vi "Smooth All Planes.vi"(8 "error in (no error)":errorcluster, 11 "Images":T1) -> (0 "error out":errorcluster, 3 "Images":T1)   [LabVIEW 2015]
uses:
  controls/Images.ctl
  <vilib>/vision/Image Controls.llb/IMAQ Image.ctl
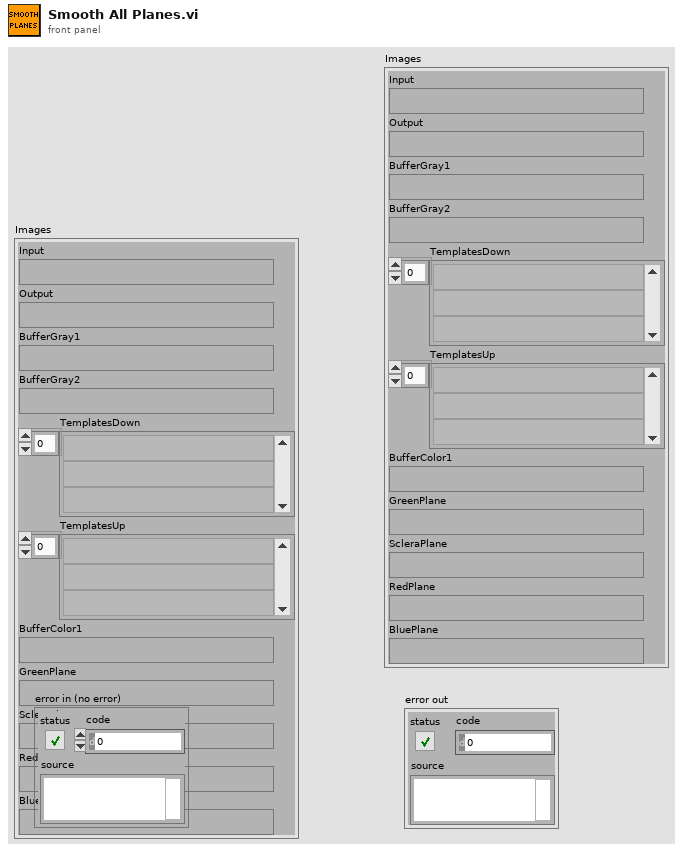
[diagram p1: front panel]
types:
  T1 = typedef "Images.ctl" = cluster{"Input":T2, "Output":T2, "BufferGray1":T2, "BufferGray2":T2, "TemplatesDown":T2[], "TemplatesUp":T2[], "BufferColor1":T2, "GreenPlane":T2, "ScleraPlane":T2, "RedPlane":T2, "BluePlane":T2}
  T2 = typedef "IMAQ Image.ctl" = refnum<image>
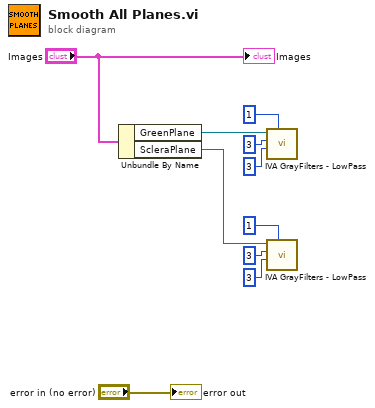
[diagram p0: block diagram]
diagram:
  n1 = Unbundle By Name("Images") -> ("GreenPlane"=w3:T2, "ScleraPlane"=w2:T2)
  n2 = call <vilib>:"IVA GrayFilters - LowPass.vi"("Tolerance"=1, "Filter size Y"=3, "Filter size X"=3, "Image In"=w3) -> ()  [unwired: 1 in, 7 out]
  n3 = call <vilib>:"IVA GrayFilters - LowPass.vi"("Tolerance"=1, "Filter size Y"=3, "Filter size X"=3, "Image In"=w2) -> ()  [unwired: 1 in, 7 out]
  "error out" <- "error in (no error)"
  "Images" <- "Images"
